vi "SpeedAccelDistanceM2.vi"(4 "Distance":u32 max=0 step=1, 5 "Immediate":u8 max=127 step=1, 6 "Accel":u32 max=127 step=1, 7 "error in (no error)":errorcluster, 8 "Address":u8, 9 "Speed":i32 max=127 step=1, 10 "VISA Refnum in":refnum<visa-resource-name>) -> (0 "error out":errorcluster, 2 "Valid":bool, 3 "VISA Refnum out":refnum<visa-resource-name>)   [LabVIEW 2015, in "Ion Motion Roboclaw.lvlib"]
uses:
  <instrlib>/Ion Motion Roboclaw/Ion Motion Roboclaw.lvlib
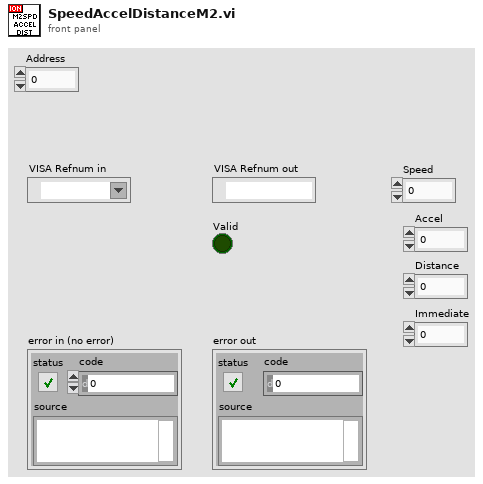
[diagram p1: front panel]
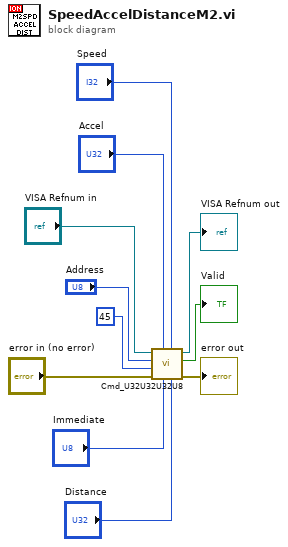
[diagram p0: block diagram]
diagram:
  n1 = call <instrlib>:"Cmd_U32U32U32U8.vi"("Arg3"="Distance", "Arg2"="Speed", "Arg4"="Immediate", "Arg1"="Accel", "error in (no error)"="error in (no error)", "Cmd"=u8 45, "Address"="Address", "VISA Refnum in"="VISA Refnum in") -> ("error out"=→"error out":errorcluster, "Valid"=→"Valid":bool, "VISA Refnum out"=→"VISA Refnum out":refnum<visa-resource-name>)  [unwired: 1 in]
